vi "partially locking read data.vi"(8 "error in":errorcluster, 9 "timeout":i32=-1, 10 "max size":i32=10000, 11 "lvlibretls connection":refnum<data-value>) -> (0 "error out":errorcluster, 2 "data":string)   [LabVIEW 2016, in "websocket upgrade handler.lvclass"]
doc: "Reads up to specified number of bytes, will usually be limited to low kb at a time."
uses:
  https/websocket/websocket upgrade handler.lvclass
  lvlibretls connection.lvclass
  lvlibretls connection.lvclass/lvlibretls connection.ctl
  tls library paths.vi
  lv tls dll.lvlib
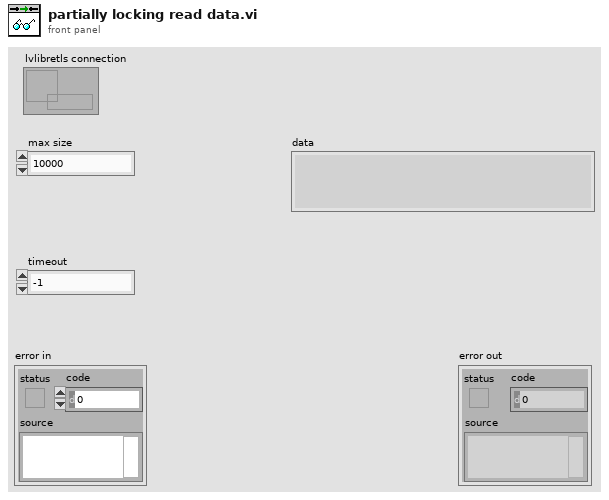
[diagram p1: front panel]
types:
  T1 = enum16{"Standard", "Buffered", "CRLF", "Immediate"}
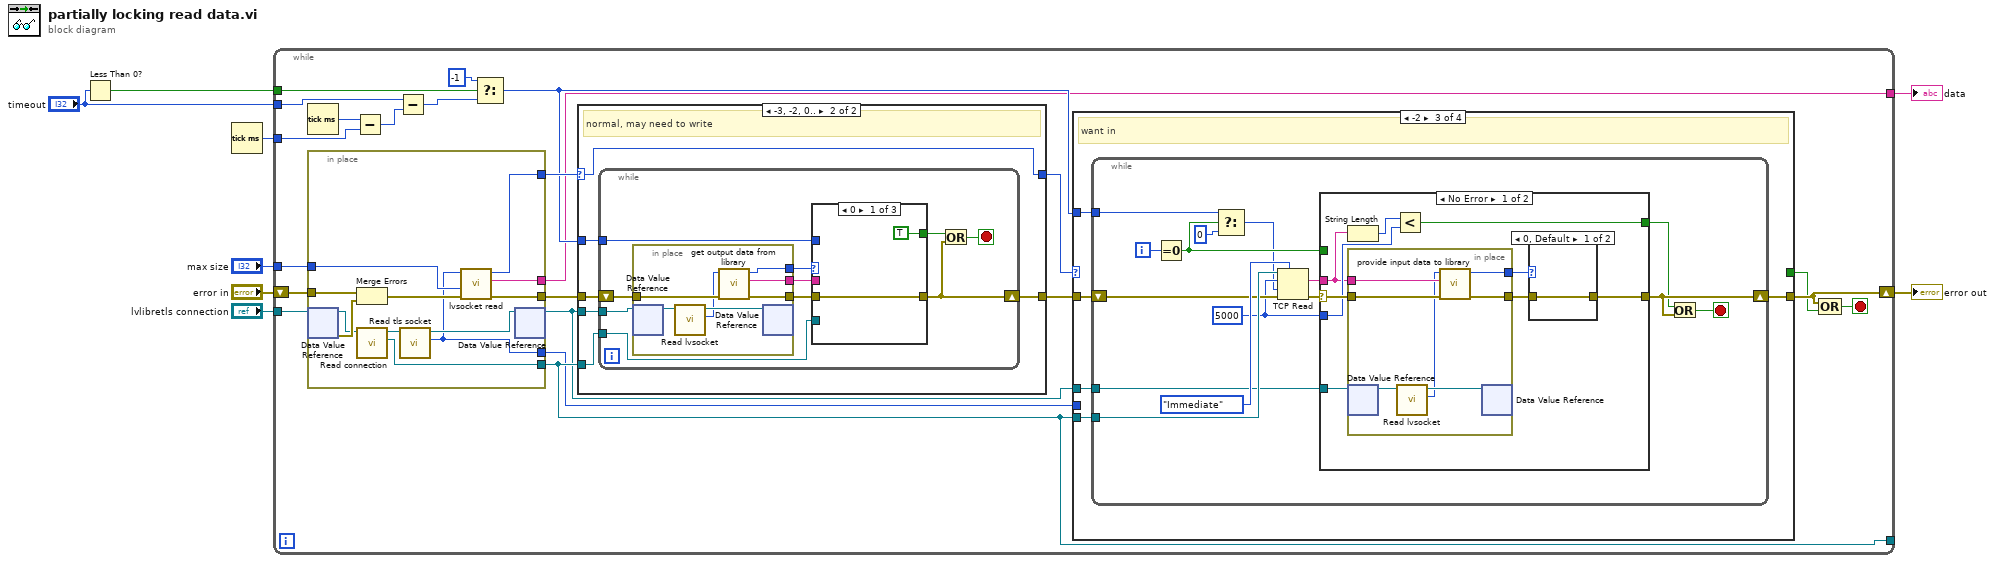
[diagram p0: block diagram]
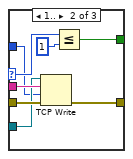
[diagram p3: hidden frame]
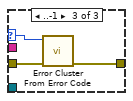
[diagram p4: hidden frame]
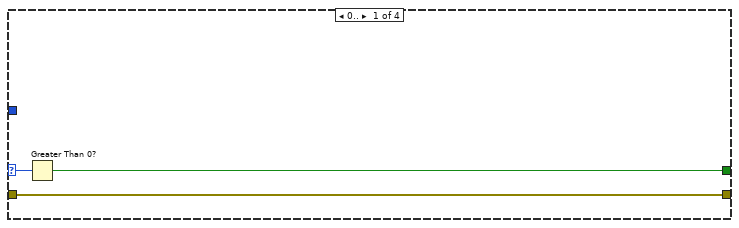
[diagram p5: hidden frame]
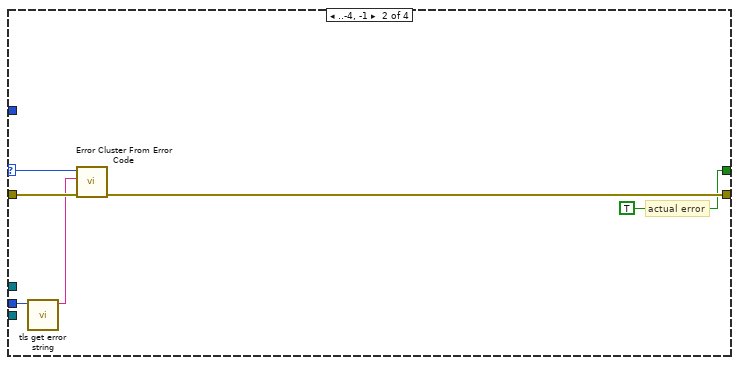
[diagram p6: hidden frame]
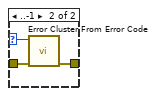
[diagram p7: hidden frame]
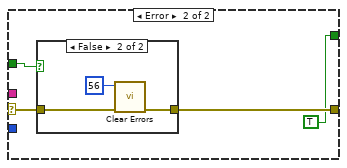
[diagram p8: hidden frame]
diagram:
  n1 = Less Than 0?(x="timeout") -> (x < 0?=w7:bool)
  n2 = Tick Count (ms)() -> (millisecond timer value=w8:u32)
  n3 = while {
    shift-right: [w29] -> w5
    shift-left: "error in" -> [w30]
    tunnel: [w11] -> _
    tunnel: "timeout" -> [w19]
    tunnel: w7 -> [w18]
    tunnel: w8 -> [w21]
    tunnel: [w14] -> w4
    tunnel: "max size" -> [w13]
    tunnel: "lvlibretls connection" -> [w12]
    stop <- w28 stop-if-true
    n4 = Tick Count (ms)() -> (millisecond timer value=w22:u32)
    n5 = in-place {
      in-place-border: w30 -> [w42]
      in-place-border: [w41] -> w26
      in-place-border: [w40] -> w23
      in-place-border: [w39] -> w14
      in-place-border: w13 -> [w38]
      in-place-border: [w32] -> w11
      in-place-border: [w31] -> w10
      n6 = in-place-dvr #1(w12) -> (w33:refnum<class "lvlibretls connection.lvclass">, w36:errorcluster)
      n7 = Merge Errors(w42, w36) -> (w37:errorcluster)
      n8 = call "Read connection.vi"("lvlibretls connection in"=w33) -> ("connection"=w32:refnum<k5>, "lvlibretls connection out"=w34:refnum<class "lvlibretls connection.lvclass">)  [unwired: 9 in]
      n9 = call "Read tls socket.vi"("lvlibretls connection in"=w34) -> ("tls socket"=w31:u64, "lvlibretls connection out"=w35:refnum<class "lvlibretls connection.lvclass">)  [unwired: 9 in]
      n10 = call "lvsocket read.vi"("error in"=w37, "max read size"=w38, "tls context"=w31) -> ("error out"=w40:errorcluster, "buffer"=w39:string, "error response"=w41:i32)  [unwired: 6 in]
      n11 = in-place-dvr #1(w35) -> (w9:refnum<data-value>)  [unwired: 1 out]
    }
    n12 = Subtract(x=w22, y=w21) -> (x-y=w20:u32)
    n13 = Subtract(x=w19, y=w20) -> (x-y=w17:i32)
    n14 = Select(t=-1, s=w18, f=w17) -> (s? t:f=w15:i32)
    n15 = case shown="-3, -2, 0.." w26 {
      selector: w26 -> [w43 w50]
      tunnel: [w43 w50] -> w25
      tunnel: [w44 w48] -> w24
      tunnel: w23 -> [w44 w49]
      tunnel: w11 -> [_ w47]
      tunnel: w15 -> [_ w46]
      tunnel: w9 -> [_ w45]
      frame Default {
      }
      frame -3, -2, 0.. {
        # "normal, may need to write"
        n16 = while {
          shift-right: [w57] -> w48
          shift-left: w49 -> [w60]
          tunnel: w47 -> [w56]
          tunnel: w46 -> [w52]
          tunnel: w45 -> [w51]
          stop <- w55 stop-if-true
          n17 = in-place {
            in-place-border: w60 -> [w67]
            in-place-border: [w66] -> w59
            in-place-border: [w65] -> w58
            in-place-border: [w64] -> w53
            n18 = in-place-dvr #2(w51) -> (w63:refnum<class "lvlibretls connection.lvclass">)  [unwired: 1 out]
            n19 = call "Read lvsocket.vi"("lvlibretls connection in"=w63) -> ("lvsocket"=w61:u64, "lvlibretls connection out"=w62:refnum<class "lvlibretls connection.lvclass">)  [unwired: 9 in]
            n20 = call "get output data from library.vi"("error in"=w67, "lvsocket"=w61) -> ("error out"=w66:errorcluster, "data"=w64:string, "err"=w65:i32)  [unwired: 7 in]
            n21 = in-place-dvr #2(w62) -> ()  [unwired: 2 out]
          }
          n22 = case shown="0" w58 {
            selector: w58 -> [_ w73 w79]
            tunnel: w59 -> [w69 w77 w80]
            tunnel: [w69 w76 w78] -> w57
            tunnel: w53 -> [_ w75 _]
            tunnel: w56 -> [_ w74 _]
            tunnel: [TRUE w71 _] -> w54
            tunnel: w52 -> [_ w70 _]
            frame 0 {
            }
            frame 1.. {
              n23 = TCP Write(connection ID=w74, data in=w75, error in (no error)=w77, 9:w70) -> (error out=w76:errorcluster)  [unwired: 2 out]
              n24 = Less Or Equal?(x=w73, y=1) -> (x <= y?=w71:bool)
            }
            frame ..-1 {
              n25 = call <vilib>:"Error Cluster From Error Code.vi"("error in (no error)"=w80, "error code (0)"=w79) -> ("error out"=w78:errorcluster)  [unwired: 7 in]
            }
          }
          n26 = Or(x=w54, y=w57) -> (x .or. y?=w55:bool)
        }
      }
    }
    n27 = case shown="-2" w25 {
      selector: w25 -> [w81 w89 _ _]
      tunnel: [w83 w88 w93 w138] -> w29
      tunnel: [w82 TRUE _ _] -> w27
      tunnel: w11 -> [_ _ w94 _]
      tunnel: w24 -> [w83 w86 w92 w138]
      tunnel: w15 -> [_ _ w91 _]
      tunnel: w10 -> [_ w85 _ _]
      tunnel: w9 -> [_ _ w90 _]
      frame 0.. {
        n28 = Greater Than 0?(x=w81) -> (x > 0?=w82:bool)
      }
      frame ..-4, -1 {
        # "actual error"
        n29 = call "tls get error string.vi"("tls context"=w85) -> ("error string"=w84:string)  [unwired: 9 in, 1 out]
        n30 = call <vilib>:"Error Cluster From Error Code.vi"("error in (no error)"=w86, "error message (\"\")"=w84, "error code (0)"=w89) -> ("error out"=w88:errorcluster)  [unwired: 6 in]
      }
      frame -2 {
        # "want in"
        n31 = while {
          tunnel: w94 -> [w109]
          shift-right: [w105] -> w93
          shift-left: w92 -> [w106]
          tunnel: w91 -> [w98]
          tunnel: w90 -> [w95]
          i -> [w104]
          stop <- w103 stop-if-true
          w101 = 5000 ("bytes to read")
          n32 = Equal To 0?(x=w104) -> (x = 0?=w99:bool)
          n33 = Select(t=w98, s=w99, f=0 ("timeout ms (25000)")) -> (s? t:f=w96:i32)
          n34 = TCP Read(connection ID=w109, bytes to read=w101, error in (no error)=w106, 7:T1."Immediate" ("mode (standard)"), 9:w96) -> (data out=w100:string, error out=w107:errorcluster)  [unwired: 1 out]
          n35 = case shown="No Error" w107 {
            selector: w107 -> [w118 w133]
            tunnel: w100 -> [w111 _]
            tunnel: [w115 w132] -> w105
            tunnel: w99 -> [_ w131]
            tunnel: [w112 TRUE] -> w102
            tunnel: w101 -> [w113 _]
            tunnel: w95 -> [w110 _]
            frame No Error {
              n36 = String Length(string=w111) -> (length=w114:i32)
              n37 = in-place {
                in-place-border: w118 -> [w125]
                in-place-border: [w124] -> w117
                in-place-border: [w123] -> w116
                in-place-border: w111 -> [w122]
                n38 = in-place-dvr #3(w110) -> (w121:refnum<class "lvlibretls connection.lvclass">)  [unwired: 1 out]
                n39 = call "Read lvsocket.vi"("lvlibretls connection in"=w121) -> ("lvsocket"=w119:u64, "lvlibretls connection out"=w120:refnum<class "lvlibretls connection.lvclass">)  [unwired: 9 in]
                n40 = call "provide input data to library.vi"("error in"=w125, "data in"=w122, "lvsocket"=w119) -> ("error out"=w124:errorcluster, "return"=w123:i32)  [unwired: 7 in]
                n41 = in-place-dvr #3(w120) -> ()  [unwired: 2 out]
              }
              n42 = Less?(x=w114, y=w113) -> (x < y?=w112:bool)
              n43 = case shown="0, Default" w116 {
                selector: w116 -> [_ w128]
                tunnel: w117 -> [w126 w129]
                tunnel: [w126 w127] -> w115
                frame 0, Default {
                }
                frame ..-1 {
                  n44 = call <vilib>:"Error Cluster From Error Code.vi"("error in (no error)"=w129, "error code (0)"=w128) -> ("error out"=w127:errorcluster)  [unwired: 7 in]
                }
              }
            }
            frame Error {
              n45 = case shown="False" w131 {
                tunnel: w133 -> [w134 w137]
                tunnel: [w134 w136] -> w132
                frame True {
                }
                frame False {
                  n46 = call <vilib>:"Clear Errors.vi"("error in (no error)"=w137, "specific error code to clear (0: all)"=56) -> ("error out"=w136:errorcluster)  [unwired: 4 in, 1 out]
                }
              }
            }
          }
          n47 = Or(x=w102, y=w105) -> (x .or. y?=w103:bool)
        }
      }
      frame -3 {
        # "want out"
      }
    }
    n48 = Compound Arithmetic op=OR(w29, w27) -> (w28:bool)
  }
  "error out" <- w5
  "data" <- w4
